vi "Read MDO waveform.vi"() -> ()   [LabVIEW 2020]
uses:
  <instrlib>/Tektronix DPO MSO 2000 4000 Series/Public/Data/Data_Low Level/Fetch Waveform (Waveform Data Type).vi
  <vilib>/Waveform/WDTFileIO.llb/Export Waveforms To Spreadsheet File (1D).vi
  <instrlib>/Tektronix DPO MSO 2000 4000 Series/Tektronix DPO MSO 2000 4000 Series.lvlib
panel:
  in  "System Array":u16[](array[ring]) items=["Channel 1", "Channel 2", "Channel 3", "Channel 4", "Math", "Reference 1", "Reference 2", "Reference 3", "Reference 4", "D0", "D1", "D2", "D3", "D4", "D5", "D6", "D7", "D8", "D9", "D10", "D11", "D12", "D13", "D14", "D15", "Amplitude", "Frequency", "Phase", "Normal", "Average", "Maximum Peak Hold", "Minimum Peak Hold"]
  out "error out":errorcluster
  out "read buffer":string
  out "Waveform Data":waveform(dbl)[](graph)
  in  "VISA resource name":refnum<visa-resource-name>
  in  "Maximum Time (10000ms)":u32=10000
  in  "error in (no error)":errorcluster
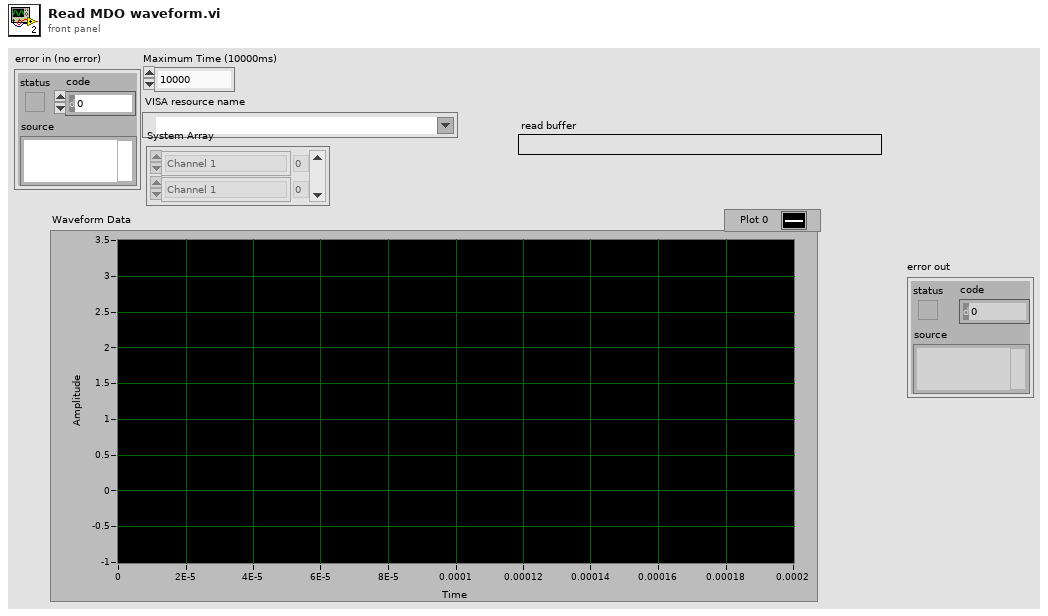
[diagram p1: front panel]
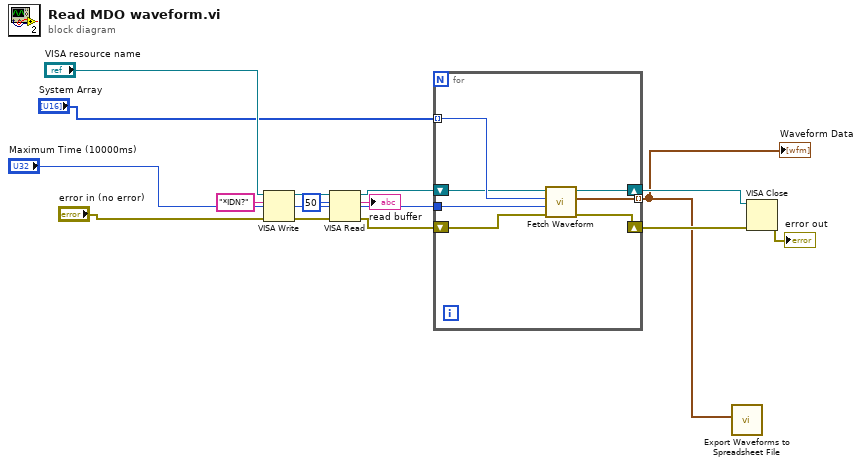
[diagram p0: block diagram]
diagram:
  n1 = VISA Write(VISA resource name="VISA resource name", write buffer="*IDN?", error in (no error)="error in (no error)") -> (VISA resource name out=w11:refnum<visa-resource-name>, error out=w14:errorcluster)  [unwired: 1 out]
  n2 = VISA Read(VISA resource name=w11, byte count=u32 50, error in (no error)=w14) -> (VISA resource name out=w9:refnum<visa-resource-name>, read buffer=→"read buffer":string, error out=w13:errorcluster)  [unwired: 1 out]
  n3 = for {
    tunnel: "Maximum Time (10000ms)" -> [w22]
    tunnel: "System Array" -> [w21] mode=indexing
    tunnel: [w20] -> w1 mode=indexing
    shift-right: [w16] -> w4
    shift-left: w13 -> [w19]
    shift-right: [w17] -> w5
    shift-left: w9 -> [w18]
    n4 = call-poly <instrlib>:"Fetch Waveform.vi"("error in (no error)"=w19, "Maximum Time (10000ms)"=w22, "Channel (0: Channel 1)"=w21, "VISA resource name"=w18) -> ("error out"=w16:errorcluster, "Waveform Data"=w20:waveform(dbl), "VISA resource name out"=w17:refnum<visa-resource-name>)  [unwired: 5 in]
  }
  "Waveform Data" <- w1
  n5 = call-poly <vilib>:"Export Waveforms to Spreadsheet File.vi"("waveforms"=w1) -> ()  [unwired: 9 in, 2 out]
  n6 = VISA Close(VISA resource name=w5, error in (no error)=w4) -> (error out=→"error out":errorcluster)
